vi "dash safety data FG.vi"(1 "Safety Data":T1, 2 "Menu":T2) -> (0 "Safety Data Out":T1)   [LabVIEW 2013]
uses:
  typedefs/fg_typedef.ctl
  typedefs/Dashboard/dashboard safety status data.ctl
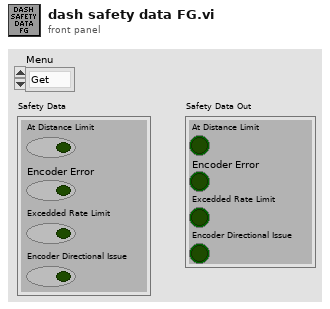
[diagram p1: front panel]
types:
  T1 = typedef "dashboard safety status data.ctl" = cluster{"At Distance Limit":bool, "Encoder Error":bool, "Excedded Rate Limit":bool, "Encoder Directional Issue":bool}
  T2 = typedef "fg_typedef.ctl" = enum16{"Get", "Set"}
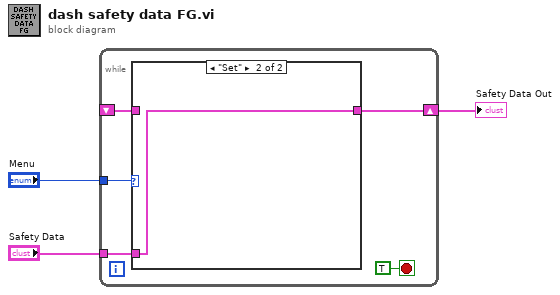
[diagram p0: block diagram]
diagram:
  n1 = while {
    tunnel: "Menu" -> [w7]
    shift-right: [w4] -> w1
    shift-left: _ -> [w6]
    tunnel: "Safety Data" -> [w5]
    stop <- TRUE stop-if-true
    n2 = case shown="\"Set\"" w7 {
      tunnel: w6 -> [w9 _]
      tunnel: [w9 w10] -> w4
      tunnel: w5 -> [_ w10]
      frame "Get", Default {
      }
      frame "Set" {
      }
    }
  }
  "Safety Data Out" <- w1
